vi "Example Clusters in ForLoop.vi"() -> ()   [LabVIEW 2014]
uses:
  <vilib>/LabVIEW Universal Transcriptor/LabVIEW to Arduino Transcriptor/Transcriptors/System API/Serial println string.vi
panel:
  out "error out":errorcluster
  in  "error in (no error)":errorcluster
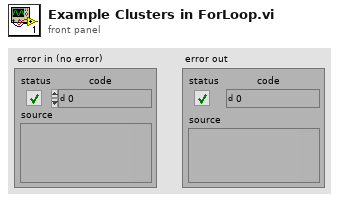
[diagram p1: front panel]
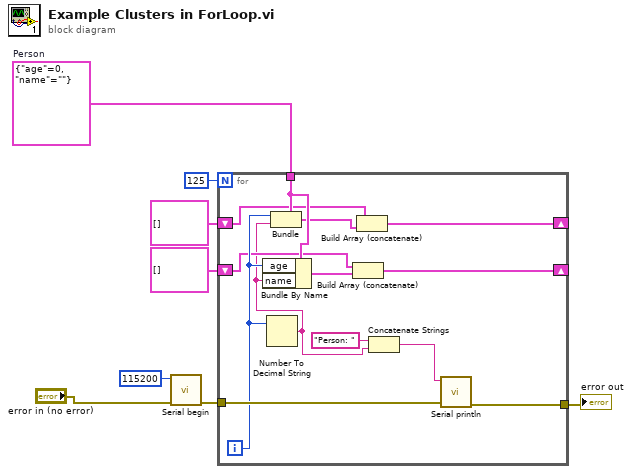
[diagram p0: block diagram]
diagram:
  w6 = cluster{"age":i32, "name":string} {"age"=0, "name"=""}  # Person
  n1 = call <vilib>:"Serial begin.vi"("Error In"="error in (no error)", "speed (Bd)"=115200) -> ("Error Out"=w7:errorcluster)  [unwired: 9 in]
  n2 = for {
    N: 125 -> [_]
    tunnel: w7 -> [w21]
    tunnel: w6 -> [w20]
    tunnel: [w19] -> w4
    shift-right: [w17] -> _
    shift-left: cluster{"age":i32, "name":string}[] [] -> [w16]
    shift-right: [w13] -> _
    shift-left: cluster{"age":i32, "name":string}[] [] -> [w12]
    i -> [w15]
    n3 = Number To Decimal String(number=w15) -> (decimal integer string=w9:string)  [unwired: 1 in]
    n4 = Bundle By Name(cluster=w20, "age"=w15, "name"=w9) -> (w14:cluster{"age":i32, "name":string})
    n5 = Bundle(cluster=w20, "age"=w15, "name"=w9) -> (w18:cluster{"age":i32, "name":string})
    n6 = Build Array (concatenate)(w12, w14) -> (w13:cluster{"age":i32, "name":string}[])
    n7 = Build Array (concatenate)(w16, w18) -> (w17:cluster{"age":i32, "name":string}[])
    n8 = Concatenate Strings("Person: " ("string"), w9) -> (w11:string)
    n9 = call-poly <vilib>:"Serial println.vi"("Error In"=w21, "string in"=w11) -> ("Error Out"=w19:errorcluster)  [unwired: 9 in]
  }
  "error out" <- w4
